vi "Read Algoparameters JSON.vi"() -> ()   [LabVIEW 2015]
uses:
  <vilib>/addons/_JKI.lib/Serialization/JSON/JKI JSON Serialization.lvlib
panel:
  out "data":T1
  out "Fault element\nJSON path":string
  in  "Algoparameters control":T1={"SpecificationVersion"="", "CompatibleSoftwareVersions"=["trt"], "AlgoParameters"={"PartsList"=[{"Name"="", "ImageStreams"=[{"ThreadName"="", "RackEnable"=FALSE, "ThreadId"=0.0, "RackId"=0.0, "DifferenceParameter"=0.0, "SplitCameraIDs"=[3], "ImagingViews"=[{"ViewName"="", "ViewEnable"=FALSE, "ImageID"=0.0, "CameraID"=0.0, "CalibrationFilePath"="", "CalibImageFormat"="", "ReferenceCoordSystem"={"Method"={"Algo"="", "BaseReference"={"OriginX"=0.0, "OriginY"=0.0, "Angle"=0.0, "AxisReference"=0.0}}, "ROI"=[{"ROI"={"Left"=0.0, "Top"=0.0, "Right"=0.0, "Bottom"=0.0, "Rotation"=0.0}, "EdgeOptions"={"EdgePolarity"=0.0, "KernelSize"=0.0, "Width"=0.0, "MinimumEdgeStrength"=0.0, "InterpolationType"=0.0, "DataProcessingMethod"=0.0}, "LineOptions"={"NumberofLines"=0.0, "Type"=0.0, "MinScore"=0.0, "MaxScore"=0.0, "Orientation"=0.0, "AngleRange"=0.0, "AngleTolerance"=0.0, "StepSize"=0.0, "MinSNR"=0.0, "MinPoints"=0.0, "HoughIterations"=0.0}, "Process"=0.0, "StepSize"=0.0, "SearchDirection"=0.0, "CircleEdgeOptions"={"SearchDirection"=0.0, "EdgeOptions"={"EdgePolarity"=0.0, "KernelSize"=0.0, "Width"=0.0, "MinimumEdgeStrength"=0.0, "InterpolationType"=0.0, "DataProcessingMethod"=0.0}}, "CircleFitOptions"={"Process"=0.0, "StepSize"=0.0, "MAxPixelRadius"=0.0}, "CircleSearchDirection"=0.0, "CurveParameters"={"ExtractionMode"=0.0, "EdgeThreshold"=0.0, "EdgeFilterSize"=0.0, "MinLength"=0.0, "RowSearchStepSize"=0.0, "ColSearchStepSize"=0.0, "MaxEndpointGap"=0.0, "Closed"=FALSE, "Subpixel"=FALSE}, "MinimumMatchScore"=0.0, "CircleDescriptor"={"MinRadius"=5.0, "MaxRadius"=0.0}, "EllipseDescriptor"={"MinMajorRadius"=0.0, "MaxMajorRadius"=0.0, "MinMinorRadius"=0.0, "MaxMinorRadius"=0.0}, "ParallelLines"={"First"=0.0, "Second"=0.0, "Third"=0.0}}], "Name"="", "OverlayOptions"={"OverlayEnable"=FALSE, "OverlayText"="", "OverlayCoords"=[5], "OverlayAngle"=0.0, "OverlayTextSize"=0.0, "OverlayTextColor"="", "OverlayROI"=FALSE, "OverlayRakeLine"=FALSE, "OverlayPoints"=FALSE}}, "CameraAngle"=[5]}]}], "Measurements"=[{"RackID"=0.0, "ImageID"=0.0, "CameraID"=0.0, "MeasurementId"=0.0, "Name"="", "AlgoName"="", "Type"="", "MeasurementEnable"=FALSE, "AlgorithmSequence"={"RefernceEdge"={"Enable"=FALSE, "Method"="", "RefROI"={"Left"=0.0, "Top"=0.0, "Right"=0.0, "Bottom"=0.0, "Rotation"=0.0}, "EdgeOptions"={"EdgePoarity"=0.0, "KernelSize"=0.0, "Width"=0.0, "MinimumEdgeStrength"=0.0, "InterpolationType"=0.0, "DataProcessingMethod"=0.0}, "LineOptions"={"NumberofLines"=0.0, "Type"=0.0, "MinScore"=0.0, "MaxScore"=0.0, "Orientation"=0.0, "AngleRange"=0.0, "AngleTolerance"=0.0, "StepSize"=0.0, "MinSNR"=0.0, "MinPoints"=0.0, "HoughIterations"=0.0}, "SearchDirection"=0.0}, "Measurement"={"ROI1"={"Enable"=FALSE, "ROI"={"Left"=0.0, "Top"=0.0, "Right"=0.0, "Bottom"=0.0, "Rotation"=0.0}, "EdgeOptions"={"EdgePoarity"=0.0, "KernelSize"=0.0, "Width"=0.0, "MinimumEdgeStrength"=0.0, "InterpolationType"=0.0, "DataProcessingMethod"=0.0}, "LineOptions"={"NumberofLines"=0.0, "Type"=0.0, "MinScore"=0.0, "MaxScore"=0.0, "Orientation"=0.0, "AngleRange"=0.0, "AngleTolerance"=0.0, "StepSize"=0.0, "MinSNR"=0.0, "MinPoints"=0.0, "HoughIterations"=0.0}, "Process"=0.0, "StepSize"=0.0, "SearchDirection"=0.0, "CircleEdgeOptions"={"SearchDirection"=0.0, "EdgeOptions"={"EdgePoarity"=0.0, "KernelSize"=0.0, "Width"=0.0, "MinimumEdgeStrength"=0.0, "InterpolationType"=0.0, "DataProcessingMethod"=0.0}}, "CircleFitOptions"={"Process"=0.0, "StepSize"=0.0, "MAxPixelRadius"=0.0}, "CircleSearchDirection"=0.0, "CurveParameters"={"ExtractionMode"=0.0, "EdgeThreshold"=0.0, "EdgeFilterSize"=0.0, "MinLength"=0.0, "RowSearchStepSize"=0.0, "ColSearchStepSize"=0.0, "MaxEndpointGap"=0.0, "Closed"=FALSE, "Subpixel"=FALSE}, "MinimumMatchScore"=0.0, "CircleDescriptor"={"MinRadius"=0.0, "MaxRadius"=0.0}, "EllipseDescriptor"={"MinMajorRadius"=0.0, "MaxMajorRadius"=0.0, "MinMinorRadius"=0.0, "MaxMinorRadius"=0.0}}, "ROI2"={"Enable"=FALSE, "ROI"={"Left"=0.0, "Top"=0.0, "Right"=0.0, "Bottom"=0.0, "Rotation"=0.0}, "EdgeOptions"={"EdgePoarity"=0.0, "KernelSize"=0.0, "Width"=0.0, "MinimumEdgeStrength"=0.0, "InterpolationType"=0.0, "DataProcessingMethod"=0.0}, "LineOptions"={"NumberofLines"=0.0, "Type"=0.0, "MinScore"=0.0, "MaxScore"=0.0, "Orientation"=0.0, "AngleRange"=0.0, "AngleTolerance"=0.0, "StepSize"=0.0, "MinSNR"=0.0, "MinPoints"=0.0, "HoughIterations"=0.0}, "Process"=0.0, "StepSize"=0.0, "SearchDirection"=0.0, "CircleEdgeOptions"={"SearchDirection"=0.0, "EdgeOptions"={"EdgePoarity"=0.0, "KernelSize"=0.0, "Width"=0.0, "MinimumEdgeStrength"=0.0, "InterpolationType"=0.0, "DataProcessingMethod"=0.0}}, "CircleFitOptions"={"Process"=0.0, "StepSize"=0.0, "MAxPixelRadius"=0.0}, "CircleSearchDirection"=0.0, "CurveParameters"={"ExtractionMode"=0.0, "EdgeThreshold"=0.0, "EdgeFilterSize"=0.0, "MinLength"=0.0, "RowSearchStepSize"=0.0, "ColSearchStepSize"=0.0, "MaxEndpointGap"=0.0, "Closed"=FALSE, "Subpixel"=FALSE}, "MinimumMatchScore"=0.0, "CircleDescriptor"={"MinRadius"=0.0, "MaxRadius"=0.0}, "EllipseDescriptor"={"MinMajorRadius"=0.0, "MaxMajorRadius"=0.0, "MinMinorRadius"=0.0, "MaxMinorRadius"=0.0}}}}, "MathExpression"={"Algorithm"="", "MathExpression"="", "ResultVariable"=""}, "MathCorrectionParameters"={"Radius"=0.0, "CurlGap"=0.0, "Thickness"=0.0, "MeasurementIndices"=[5], "MathAlgoName"="", "MathAlgoFormula"="", "CorrectionForAngle"=[35], "NumericAray"=[0], "StringArray"=["gfdgf"]}, "ResultVariableCluster"={"RVName"="", "RVSequence"="", "RVIndex"=0.0, "RVID"=0.0, "RVValue"=0.0}, "CalibrationCoefficients"={"A1"=0.0, "A2"=0.0, "A3"=0.0}, "UserCalibCoefficients"={"UserCorrectionLinearityCoeff"=0.0, "UserCorrectionBiasCoeff"=0.0}, "SpecValues"={"LCL"=0.0, "UCL"=0.0, "LSL"=0.0, "USL"=0.0, "NominalValue"=0.0}, "OverlayOptions"={"OverlayEnable"=FALSE, "OverlayText"="", "OverlayCoords"=[3], "OverlayAngle"=0.0, "OverlayTextSize"=0.0, "OverlayTextColor"="", "OverlayROI"=FALSE, "OverlayRakeLine"=FALSE, "OverlayPoints"=FALSE}, "DatalogEnable"=FALSE, "DisplayIcon"="test"}]}], "AlgoDefaultParameters"={"AlgoName"="", "Enable"=FALSE, "AlgorithmSequenceDefault"={"RefernceEdgeDefault"={"Method"="", "RefROI"={"Left"=0.0, "Top"=0.0, "Right"=0.0, "Bottom"=0.0, "Rotation"=0.0}, "EdgeOptions"={"EdgePoarity"=0.0, "KernelSize"=0.0, "Width"=0.0, "MinimumEdgeStrength"=0.0, "InterpolationType"=0.0, "DataProcessingMethod"=0.0}, "LineOptions"={"NumberofLines"=0.0, "Type"=0.0, "MinScore"=0.0, "MaxScore"=0.0, "Orientation"=0.0, "AngleRange"=0.0, "AngleTolerance"=0.0, "StepSize"=0.0, "MinSNR"=0.0, "MinPoints"=0.0, "HoughIterations"=0.0}, "SearchDirection"=0.0}, "MeasurementDefault"={"ROI1"={"ROI"={"Left"=0.0, "Top"=0.0, "Right"=0.0, "Bottom"=0.0, "Rotation"=0.0}, "EdgeOptions"={"EdgePoarity"=0.0, "KernelSize"=0.0, "Width"=0.0, "MinimumEdgeStrength"=0.0, "InterpolationType"=0.0, "DataProcessingMethod"=0.0}, "LineOptions"={"NumberofLines"=0.0, "Type"=0.0, "MinScore"=0.0, "MaxScore"=0.0, "Orientation"=0.0, "AngleRange"=0.0, "AngleTolerance"=0.0, "StepSize"=0.0, "MinSNR"=0.0, "MinPoints"=0.0, "HoughIterations"=0.0}, "Process"=0.0, "StepSize"=0.0, "SearchDirection"=0.0, "CircleEdgeOptions"={"SearchDirection"=0.0, "EdgeOptions"={"EdgePoarity"=0.0, "KernelSize"=0.0, "Width"=0.0, "MinimumEdgeStrength"=0.0, "InterpolationType"=0.0, "DataProcessingMethod"=0.0}}, "CircleFitOptions"={"Process"=0.0, "StepSize"=0.0, "MAxPixelRadius"=0.0}, "CircleSearchDirection"=0.0, "CurveParameters"={"ExtractionMode"=0.0, "EdgeThreshold"=0.0, "EdgeFilterSize"=0.0, "MinLength"=0.0, "RowSearchStepSize"=0.0, "ColSearchStepSize"=0.0, "MaxEndpointGap"=0.0, "Closed"=0.0, "Subpixel"=0.0}, "MinimumMatchScore"=0.0, "CircleDescriptor"={"MinRadius"=0.0, "MaxRadius"=0.0}, "EllipseDescriptor"={"MinMajorRadius"=0.0, "MaxMajorRadius"=0.0, "MinMinorRadius"=0.0, "MaxMinorRadius"=0.0}, "OverlayOptions"={"OverlayEnable"=FALSE, "OverlayText"="", "OverlayCoords"=[34], "OverlayAngle"=0.0, "OverlayTextSize"=0.0, "OverlayTextColor"=""}, "ResultVariable"=""}, "ROI2"={"ROI"={"Left"=0.0, "Top"=0.0, "Right"=0.0, "Bottom"=0.0, "Rotation"=0.0}, "EdgeOptions"={"EdgePoarity"=0.0, "KernelSize"=0.0, "Width"=0.0, "MinimumEdgeStrength"=0.0, "InterpolationType"=0.0, "DataProcessingMethod"=0.0}, "LineOptions"={"NumberofLines"=0.0, "Type"=0.0, "MinScore"=0.0, "MaxScore"=0.0, "Orientation"=0.0, "AngleRange"=0.0, "AngleTolerance"=0.0, "StepSize"=0.0, "MinSNR"=0.0, "MinPoints"=0.0, "HoughIterations"=0.0}, "Process"=0.0, "StepSize"=0.0, "SearchDirection"=0.0, "CircleEdgeOptions"={"SearchDirection"=0.0, "EdgeOptions"={"EdgePoarity"=0.0, "KernelSize"=0.0, "Width"=0.0, "MinimumEdgeStrength"=0.0, "InterpolationType"=0.0, "DataProcessingMethod"=0.0}}, "CircleFitOptions"={"Process"=0.0, "StepSize"=0.0, "MaxPixelRadius"=0.0}, "CircleSearchDirection"=0.0, "CurveParameters"={"ExtractionMode"=0.0, "EdgeThreshold"=0.0, "EdgeFilterSize"=0.0, "MinLength"=0.0, "RowSearchStepSize"=0.0, "ColSearchStepSize"=0.0, "MaxEndpointGap"=0.0, "Closed"=0.0, "Subpixel"=0.0}, "MinimumMatchScore"=0.0, "CircleDescriptor"={"MinRadius"=0.0, "MaxRadius"=0.0}, "EllipseDescriptor"={"MinMajorRadius"=0.0, "MaxMajorRadius"=0.0, "MinMinorRadius"=0.0, "MaxMinorRadius"=0.0}, "OverlayOptions"={"OverlayEnable"=FALSE, "OverlayText"="", "OverlayCoords"=[23], "OverlayAngle"=0.0, "OverlayTextSize"=0.0, "OverlayTextColor"=""}, "ResultVariable"=""}}, "MathExpressionDefault"={"Algorithm"="", "MathExpression"="", "ResultVariable"=""}}, "CalibrationCoefficients"={"A1"=0.0, "A2"=0.0, "A3"=0.0}, "UserCalibCoefficients"={"UserCorrectionBiasCoeff"=0.0, "UserCorrectionLinearityCoeff"=0.0}, "OverlayOptions"={"OverlayEnable"=FALSE, "OverlayText"="", "OverlayCoords"=[43], "OverlayAngle"=0.0, "OverlayTextSize"=0.0, "OverlayTextColor"=""}, "DatalogEnable"=FALSE, "DisplayIcon"=""}}}
  out "Output JSON string":string
  out "error out":errorcluster
  in  "error in (no error)":errorcluster
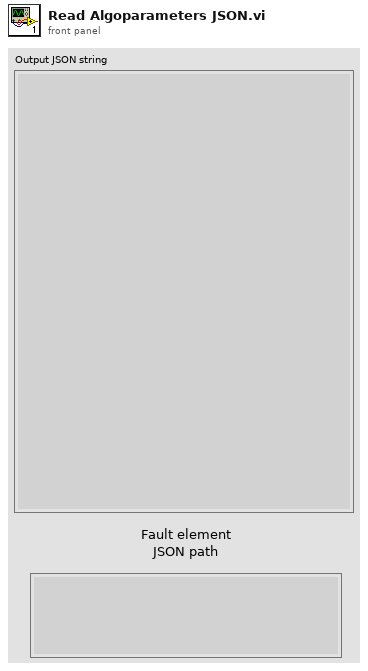
[diagram p1: front panel]
types:
  T1 = cluster{"SpecificationVersion":string, "CompatibleSoftwareVersions":string[], "AlgoParameters":cluster{"PartsList":cluster{"Name":string, "ImageStreams":cluster{"ThreadName":string, "RackEnable":bool, "ThreadId":dbl, "RackId":dbl, "DifferenceParameter":dbl, "SplitCameraIDs":i32[], "ImagingViews":cluster{"ViewName":string, "ViewEnable":bool, "ImageID":dbl, "CameraID":dbl, "CalibrationFilePath":string, "CalibImageFormat":string, "ReferenceCoordSystem":cluster{"Method":cluster{"Algo":string, "BaseReference":cluster{"OriginX":dbl, "OriginY":dbl, "Angle":dbl, "AxisReference":dbl}}, "ROI":cluster{"ROI":cluster{"Left":dbl, "Top":dbl, "Right":dbl, "Bottom":dbl, "Rotation":dbl}, "EdgeOptions":cluster{"EdgePolarity":dbl, "KernelSize":dbl, "Width":dbl, "MinimumEdgeStrength":dbl, "InterpolationType":dbl, "DataProcessingMethod":dbl}, "LineOptions":cluster{"NumberofLines":dbl, "Type":dbl, "MinScore":dbl, "MaxScore":dbl, "Orientation":dbl, "AngleRange":dbl, "AngleTolerance":dbl, "StepSize":dbl, "MinSNR":dbl, "MinPoints":dbl, "HoughIterations":dbl}, "Process":dbl, "StepSize":dbl, "SearchDirection":dbl, "CircleEdgeOptions":cluster{"SearchDirection":dbl, "EdgeOptions":cluster{"EdgePolarity":dbl, "KernelSize":dbl, "Width":dbl, "MinimumEdgeStrength":dbl, "InterpolationType":dbl, "DataProcessingMethod":dbl}}, "CircleFitOptions":cluster{"Process":dbl, "StepSize":dbl, "MAxPixelRadius":dbl}, "CircleSearchDirection":dbl, "CurveParameters":cluster{"ExtractionMode":dbl, "EdgeThreshold":dbl, "EdgeFilterSize":dbl, "MinLength":dbl, "RowSearchStepSize":dbl, "ColSearchStepSize":dbl, "MaxEndpointGap":dbl, "Closed":bool, "Subpixel":bool}, "MinimumMatchScore":dbl, "CircleDescriptor":cluster{"MinRadius":dbl, "MaxRadius":dbl}, "EllipseDescriptor":cluster{"MinMajorRadius":dbl, "MaxMajorRadius":dbl, "MinMinorRadius":dbl, "MaxMinorRadius":dbl}, "ParallelLines":cluster{"First":dbl, "Second":dbl, "Third":dbl}}[], "Name":string, "OverlayOptions":cluster{"OverlayEnable":bool, "OverlayText":string, "OverlayCoords":i32[], "OverlayAngle":dbl, "OverlayTextSize":dbl, "OverlayTextColor":string, "OverlayROI":bool, "OverlayRakeLine":bool, "OverlayPoints":bool}}, "CameraAngle":i32[]}[]}[], "Measurements":cluster{"RackID":dbl, "ImageID":dbl, "CameraID":dbl, "MeasurementId":dbl, "Name":string, "AlgoName":string, "Type":string, "MeasurementEnable":bool, "AlgorithmSequence":cluster{"RefernceEdge":cluster{"Enable":bool, "Method":string, "RefROI":cluster{"Left":dbl, "Top":dbl, "Right":dbl, "Bottom":dbl, "Rotation":dbl}, "EdgeOptions":cluster{"EdgePoarity":dbl, "KernelSize":dbl, "Width":dbl, "MinimumEdgeStrength":dbl, "InterpolationType":dbl, "DataProcessingMethod":dbl}, "LineOptions":cluster{"NumberofLines":dbl, "Type":dbl, "MinScore":dbl, "MaxScore":dbl, "Orientation":dbl, "AngleRange":dbl, "AngleTolerance":dbl, "StepSize":dbl, "MinSNR":dbl, "MinPoints":dbl, "HoughIterations":dbl}, "SearchDirection":dbl}, "Measurement":cluster{"ROI1":cluster{"Enable":bool, "ROI":cluster{"Left":dbl, "Top":dbl, "Right":dbl, "Bottom":dbl, "Rotation":dbl}, "EdgeOptions":cluster{"EdgePoarity":dbl, "KernelSize":dbl, "Width":dbl, "MinimumEdgeStrength":dbl, "InterpolationType":dbl, "DataProcessingMethod":dbl}, "LineOptions":cluster{"NumberofLines":dbl, "Type":dbl, "MinScore":dbl, "MaxScore":dbl, "Orientation":dbl, "AngleRange":dbl, "AngleTolerance":dbl, "StepSize":dbl, "MinSNR":dbl, "MinPoints":dbl, "HoughIterations":dbl}, "Process":dbl, "StepSize":dbl, "SearchDirection":dbl, "CircleEdgeOptions":cluster{"SearchDirection":dbl, "EdgeOptions":cluster{"EdgePoarity":dbl, "KernelSize":dbl, "Width":dbl, "MinimumEdgeStrength":dbl, "InterpolationType":dbl, "DataProcessingMethod":dbl}}, "CircleFitOptions":cluster{"Process":dbl, "StepSize":dbl, "MAxPixelRadius":dbl}, "CircleSearchDirection":dbl, "CurveParameters":cluster{"ExtractionMode":dbl, "EdgeThreshold":dbl, "EdgeFilterSize":dbl, "MinLength":dbl, "RowSearchStepSize":dbl, "ColSearchStepSize":dbl, "MaxEndpointGap":dbl, "Closed":bool, "Subpixel":bool}, "MinimumMatchScore":dbl, "CircleDescriptor":cluster{"MinRadius":dbl, "MaxRadius":dbl}, "EllipseDescriptor":cluster{"MinMajorRadius":dbl, "MaxMajorRadius":dbl, "MinMinorRadius":dbl, "MaxMinorRadius":dbl}}, "ROI2":cluster{"Enable":bool, "ROI":cluster{"Left":dbl, "Top":dbl, "Right":dbl, "Bottom":dbl, "Rotation":dbl}, "EdgeOptions":cluster{"EdgePoarity":dbl, "KernelSize":dbl, "Width":dbl, "MinimumEdgeStrength":dbl, "InterpolationType":dbl, "DataProcessingMethod":dbl}, "LineOptions":cluster{"NumberofLines":dbl, "Type":dbl, "MinScore":dbl, "MaxScore":dbl, "Orientation":dbl, "AngleRange":dbl, "AngleTolerance":dbl, "StepSize":dbl, "MinSNR":dbl, "MinPoints":dbl, "HoughIterations":dbl}, "Process":dbl, "StepSize":dbl, "SearchDirection":dbl, "CircleEdgeOptions":cluster{"SearchDirection":dbl, "EdgeOptions":cluster{"EdgePoarity":dbl, "KernelSize":dbl, "Width":dbl, "MinimumEdgeStrength":dbl, "InterpolationType":dbl, "DataProcessingMethod":dbl}}, "CircleFitOptions":cluster{"Process":dbl, "StepSize":dbl, "MAxPixelRadius":dbl}, "CircleSearchDirection":dbl, "CurveParameters":cluster{"ExtractionMode":dbl, "EdgeThreshold":dbl, "EdgeFilterSize":dbl, "MinLength":dbl, "RowSearchStepSize":dbl, "ColSearchStepSize":dbl, "MaxEndpointGap":dbl, "Closed":bool, "Subpixel":bool}, "MinimumMatchScore":dbl, "CircleDescriptor":cluster{"MinRadius":dbl, "MaxRadius":dbl}, "EllipseDescriptor":cluster{"MinMajorRadius":dbl, "MaxMajorRadius":dbl, "MinMinorRadius":dbl, "MaxMinorRadius":dbl}}}}, "MathExpression":cluster{"Algorithm":string, "MathExpression":string, "ResultVariable":string}, "MathCorrectionParameters":cluster{"Radius":dbl, "CurlGap":dbl, "Thickness":dbl, "MeasurementIndices":i32[], "MathAlgoName":string, "MathAlgoFormula":string, "CorrectionForAngle":i32[], "NumericAray":i32[], "StringArray":string[]}, "ResultVariableCluster":cluster{"RVName":string, "RVSequence":string, "RVIndex":dbl, "RVID":dbl, "RVValue":dbl}, "CalibrationCoefficients":cluster{"A1":dbl, "A2":dbl, "A3":dbl}, "UserCalibCoefficients":cluster{"UserCorrectionLinearityCoeff":dbl, "UserCorrectionBiasCoeff":dbl}, "SpecValues":cluster{"LCL":dbl, "UCL":dbl, "LSL":dbl, "USL":dbl, "NominalValue":dbl}, "OverlayOptions":cluster{"OverlayEnable":bool, "OverlayText":string, "OverlayCoords":i32[], "OverlayAngle":dbl, "OverlayTextSize":dbl, "OverlayTextColor":string, "OverlayROI":bool, "OverlayRakeLine":bool, "OverlayPoints":bool}, "DatalogEnable":bool, "DisplayIcon":string}[]}[], "AlgoDefaultParameters":cluster{"AlgoName":string, "Enable":bool, "AlgorithmSequenceDefault":cluster{"RefernceEdgeDefault":cluster{"Method":string, "RefROI":cluster{"Left":dbl, "Top":dbl, "Right":dbl, "Bottom":dbl, "Rotation":dbl}, "EdgeOptions":cluster{"EdgePoarity":dbl, "KernelSize":dbl, "Width":dbl, "MinimumEdgeStrength":dbl, "InterpolationType":dbl, "DataProcessingMethod":dbl}, "LineOptions":cluster{"NumberofLines":dbl, "Type":dbl, "MinScore":dbl, "MaxScore":dbl, "Orientation":dbl, "AngleRange":dbl, "AngleTolerance":dbl, "StepSize":dbl, "MinSNR":dbl, "MinPoints":dbl, "HoughIterations":dbl}, "SearchDirection":dbl}, "MeasurementDefault":cluster{"ROI1":cluster{"ROI":cluster{"Left":dbl, "Top":dbl, "Right":dbl, "Bottom":dbl, "Rotation":dbl}, "EdgeOptions":cluster{"EdgePoarity":dbl, "KernelSize":dbl, "Width":dbl, "MinimumEdgeStrength":dbl, "InterpolationType":dbl, "DataProcessingMethod":dbl}, "LineOptions":cluster{"NumberofLines":dbl, "Type":dbl, "MinScore":dbl, "MaxScore":dbl, "Orientation":dbl, "AngleRange":dbl, "AngleTolerance":dbl, "StepSize":dbl, "MinSNR":dbl, "MinPoints":dbl, "HoughIterations":dbl}, "Process":dbl, "StepSize":dbl, "SearchDirection":dbl, "CircleEdgeOptions":cluster{"SearchDirection":dbl, "EdgeOptions":cluster{"EdgePoarity":dbl, "KernelSize":dbl, "Width":dbl, "MinimumEdgeStrength":dbl, "InterpolationType":dbl, "DataProcessingMethod":dbl}}, "CircleFitOptions":cluster{"Process":dbl, "StepSize":dbl, "MAxPixelRadius":dbl}, "CircleSearchDirection":dbl, "CurveParameters":cluster{"ExtractionMode":dbl, "EdgeThreshold":dbl, "EdgeFilterSize":dbl, "MinLength":dbl, "RowSearchStepSize":dbl, "ColSearchStepSize":dbl, "MaxEndpointGap":dbl, "Closed":dbl, "Subpixel":dbl}, "MinimumMatchScore":dbl, "CircleDescriptor":cluster{"MinRadius":dbl, "MaxRadius":dbl}, "EllipseDescriptor":cluster{"MinMajorRadius":dbl, "MaxMajorRadius":dbl, "MinMinorRadius":dbl, "MaxMinorRadius":dbl}, "OverlayOptions":cluster{"OverlayEnable":bool, "OverlayText":string, "OverlayCoords":i32[], "OverlayAngle":dbl, "OverlayTextSize":dbl, "OverlayTextColor":string}, "ResultVariable":string}, "ROI2":cluster{"ROI":cluster{"Left":dbl, "Top":dbl, "Right":dbl, "Bottom":dbl, "Rotation":dbl}, "EdgeOptions":cluster{"EdgePoarity":dbl, "KernelSize":dbl, "Width":dbl, "MinimumEdgeStrength":dbl, "InterpolationType":dbl, "DataProcessingMethod":dbl}, "LineOptions":cluster{"NumberofLines":dbl, "Type":dbl, "MinScore":dbl, "MaxScore":dbl, "Orientation":dbl, "AngleRange":dbl, "AngleTolerance":dbl, "StepSize":dbl, "MinSNR":dbl, "MinPoints":dbl, "HoughIterations":dbl}, "Process":dbl, "StepSize":dbl, "SearchDirection":dbl, "CircleEdgeOptions":cluster{"SearchDirection":dbl, "EdgeOptions":cluster{"EdgePoarity":dbl, "KernelSize":dbl, "Width":dbl, "MinimumEdgeStrength":dbl, "InterpolationType":dbl, "DataProcessingMethod":dbl}}, "CircleFitOptions":cluster{"Process":dbl, "StepSize":dbl, "MaxPixelRadius":dbl}, "CircleSearchDirection":dbl, "CurveParameters":cluster{"ExtractionMode":dbl, "EdgeThreshold":dbl, "EdgeFilterSize":dbl, "MinLength":dbl, "RowSearchStepSize":dbl, "ColSearchStepSize":dbl, "MaxEndpointGap":dbl, "Closed":dbl, "Subpixel":dbl}, "MinimumMatchScore":dbl, "CircleDescriptor":cluster{"MinRadius":dbl, "MaxRadius":dbl}, "EllipseDescriptor":cluster{"MinMajorRadius":dbl, "MaxMajorRadius":dbl, "MinMinorRadius":dbl, "MaxMinorRadius":dbl}, "OverlayOptions":cluster{"OverlayEnable":bool, "OverlayText":string, "OverlayCoords":i32[], "OverlayAngle":dbl, "OverlayTextSize":dbl, "OverlayTextColor":string}, "ResultVariable":string}}, "MathExpressionDefault":cluster{"Algorithm":string, "MathExpression":string, "ResultVariable":string}}, "CalibrationCoefficients":cluster{"A1":dbl, "A2":dbl, "A3":dbl}, "UserCalibCoefficients":cluster{"UserCorrectionBiasCoeff":dbl, "UserCorrectionLinearityCoeff":dbl}, "OverlayOptions":cluster{"OverlayEnable":bool, "OverlayText":string, "OverlayCoords":i32[], "OverlayAngle":dbl, "OverlayTextSize":dbl, "OverlayTextColor":string}, "DatalogEnable":bool, "DisplayIcon":string}}}
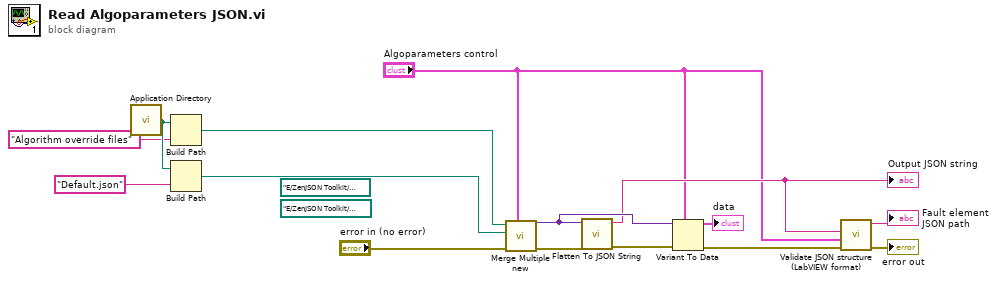
[diagram p0: block diagram]
diagram:
  (unwired) path "E:/ZenJSON Toolkit/Developer files/JSON modifications demo/Algorithm JSON testing/Algorithm default.txt" ("Default JSON filepath")
  (unwired) path "E:/ZenJSON Toolkit/Developer files/JSON modifications demo/Algorithm JSON testing/Algorithm override files" ("Merging folder filepath")
  n1 = call <vilib>:"Application Directory.vi"() -> ("Application Directory"=w5:path)
  n2 = Build Path(base path=w5, name or relative path="Algorithm override files") -> (appended path=w2:path)
  n3 = Build Path(base path=w5, name or relative path="Default.json") -> (appended path=w1:path)
  n4 = call "Merge Multiple new.vi"("Reference Variant"="Algoparameters control", "error in (no error)"="error in (no error)", "Default JSON filepath"=w1, "Merging folder filepath"=w2) -> ("error out"=w14:errorcluster, "Output Merged Cluster"=w13:variant)  [unwired: 6 in]
  n5 = call <vilib>:"Flatten To JSON String.vi"("error in (no error)"=w14, "Variant"=w13) -> ("error out"=w12:errorcluster, "JSON String"=w8:string)  [unwired: 8 in]
  "Output JSON string" <- w8
  n6 = Variant To Data(error in=w12, type="Algoparameters control", Variant=w13) -> (data=→"data":T1, error out=w9:errorcluster)
  n7 = call "Validate JSON structure (LabVIEW format).vi"("error in (no error)"=w9, "Reference cluster"="Algoparameters control", "Compare structure"=w8) -> ("error out"=→"error out":errorcluster, "Fault element\nJSON path"=→"Fault element\nJSON path":string)  [unwired: 7 in]
